vi "MTM2_getSample_netMomentsTotal.vi"(8 "error in (no error)":errorcluster, 11 "netMomentsTotal_Ctl":T1) -> (0 "error out":errorcluster, 2 "function return":i32, 3 "netMomentsTotal_Ctl out":T1)   [LabVIEW 2018, in "SALLV_MTM2.lvlib"]
doc: "int MTM2_shm_getSample_netMomentsTotalLV(MTM2_netMomentsTotalLV *netMomentsTotal_Ctl );"
uses:
  DataTypes/netMomentsTotal.ctl
  SALLV_MTM2.lvlib
  SALLV_MTM2.so
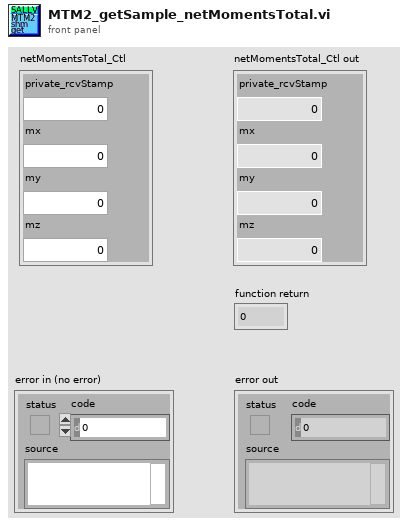
[diagram p1: front panel]
types:
  T1 = typedef "SALLV_MTM2.lvlib/netMomentsTotal.ctl" = cluster{"private_rcvStamp":dbl, "mx":dbl, "my":dbl, "mz":dbl}
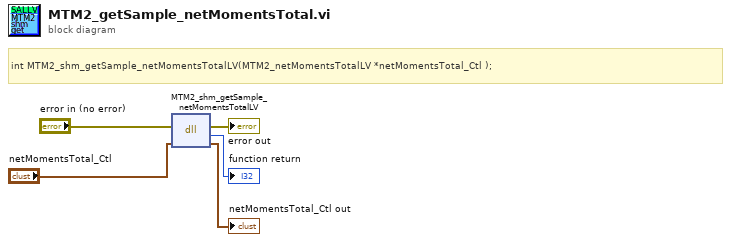
[diagram p0: block diagram]
diagram:
  # "int MTM2_shm_getSample_netMomentsTotalLV(MTM2_netMomentsTotalLV *netMomentsTotal_Ctl );"
  n1 = dll-call lib="home/ttsai/Documents/salTestLabViewApi/SALLV_MTM2/SALLV_MTM2.*" fn="MTM2_shm_getSample_netMomentsTotalLV"(error in="error in (no error)", "netMomentsTotal_Ctl"="netMomentsTotal_Ctl") -> (error out=→"error out":errorcluster, →"function return":i32, "netMomentsTotal_Ctl"=→"netMomentsTotal_Ctl out":T1)  [unwired: 2 in, 1 out]
